vi "DAQ - Set Recording Length.vi"(0 "reference in":refnum<class "GSwFormDSP.lvclass">, 5 "error in (no error)":errorcluster, 7 "DAQ.Duration (sec)":dbl) -> (14 "reference out":refnum<class "GSwFormDSP.lvclass">, 19 "error out":errorcluster)   [LabVIEW 2020, in "GSwFormDSP.lvclass"]
uses:
  GSwFormDSP.lvclass
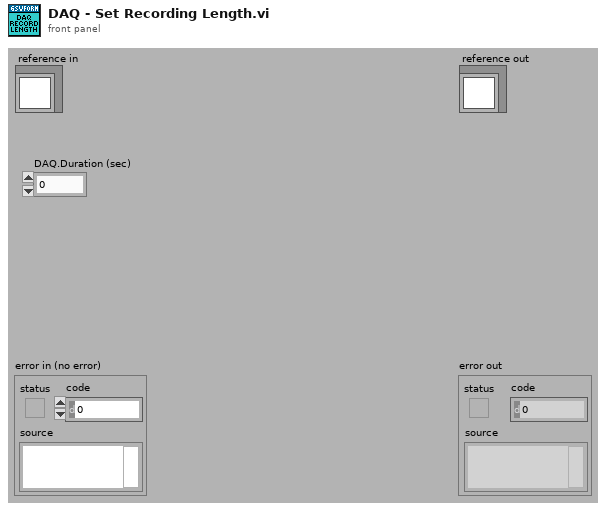
[diagram p1: front panel]
types:
  T1 = typedef "GSwFormDSP.lvclass/ObjectAttributesRef.ctl" = refnum<data-value>
  T2 = typedef "GSwFormDSP.lvclass/ObjectAttributes.ctl" = cluster{"Wform Ref":refnum<data-value>, "Nb Signals":i32, "Spectral Function Parameters":T3, "FFT":waveform(cdb)[], "Nb FFT":i32, "Nb Averages":i32[], "Reference Indexes":i32[], "Response Indexes":i32[], "Coherence":waveform(dbl)[], "TDF Parameters":T5, "DAQ":cluster{"Duration (sec)":dbl, "Buffer Size (Samples)":i32, "Offset (Samples)":i32}, "Filter Impulse Response (TDF)":waveform(dbl), "Sound Playback":T6}
  T3 = typedef "GSwFormDSP.lvclass/Spectral Parameters.ctl" = cluster{"Frequency resolution (Hz)":dbl, "Overlap":dbl, "Window":T4}
  T4 = typedef "NI_AALPro.lvlib/windowTd.ctl" = u32
  T5 = typedef "GSwFormDSP.lvclass/TDF Parameters.ctl" = cluster{"Filter":enum32{"Lowpass", "Highpass", "Bandpass", "Bandstop"}, "Type:":enum16{"Butterworth", "Chebyshev", "Inv Chebyshev", "Elliptic", "Bessel"}, "LP cutoff freq":dbl, "HP cutoff freq":dbl, "Order":i32, "passband ripple (dB)":dbl, "stopband attenuation (dB)":dbl, "Phaseless Filter":bool, "Include Fade IN and OUT":bool}
  T6 = typedef "GSwFormDSP.lvclass/Sound Playback.ctl" = cluster{"Timer start (ms)":u32, "task ID":T7, "Cursor Init Location (s)":dbl, "SC Volume":dbl}
  T7 = typedef "Sound Output Task ID.ctl" = u32
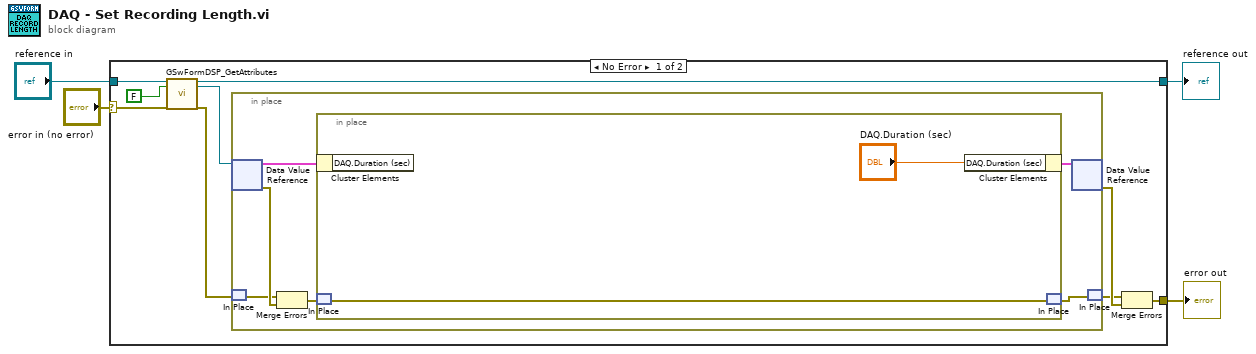
[diagram p0: block diagram]
diagram:
  n1 = case shown="No Error" "error in (no error)" {
    selector: "error in (no error)" -> [w9 w23]
    tunnel: [w13 w23] -> w3
    tunnel: [w8 w22] -> w1
    tunnel: "reference in" -> [w11 w22]
    frame No Error {
      n2 = call "GSwFormDSP_GetAttributes.vi"("reference in"=w11, "return data? (T)"=FALSE, "error in (no error)"=w9) -> ("reference out"=w8:refnum<class "GSwFormDSP.lvclass">, "attributes ref"=w7:T1, "error out"=w6:errorcluster)  [unwired: 13 in, 1 out]
      n3 = in-place {
        n4 = in-place-dvr #1(w7) -> (w18:T2, w17:errorcluster)
        n5 = in-place-match #2(w6) -> (w16:errorcluster)
        n6 = Merge Errors(w16, w17) -> (w15:errorcluster)
        n7 = in-place {
          n8 = in-place-cluster #3(w18) -> ()  [unwired: 1 out]
          n9 = in-place-match #4(w15) -> (w21:errorcluster)
          n10 = in-place-cluster #3("DAQ.Duration (sec)"="DAQ.Duration (sec)") -> (w19:T2)
          n11 = in-place-match #4(w21) -> (w14:errorcluster)
        }
        n12 = in-place-dvr #1(w19) -> (w12:errorcluster)  [unwired: 1 out]
        n13 = in-place-match #2(w14) -> (w5:errorcluster)
      }
      n14 = Merge Errors(w5, w12) -> (w13:errorcluster)
    }
    frame Error {
    }
  }
  "error out" <- w3
  "reference out" <- w1
